vi "GetHandleBySerial.vi"(1 "Serial Number":i16) -> (0 "Handle":i32)   [LabVIEW 2012]
uses:
  Madlib.dll
panel:
  # "Acquires a handle to a specific device. Can be\nused as a subVI."
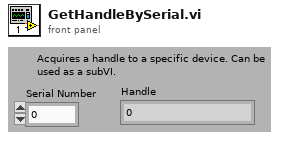
[diagram p1: front panel]
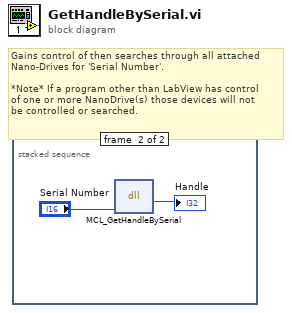
[diagram p0: block diagram]
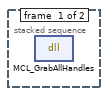
[diagram p2: hidden frame]
diagram:
  # "Gains control of then searches through all attached\nNano-Drives for 'Serial Number'.\n\n*Note* If a program other than LabView has control\nof one or more NanoDrive(s) those devices will not\nbe controlled or searched."
  n1 = stacked-sequence {
    frame #0 {
      n2 = dll-call lib="C:/Users/Labview/Desktop/SRR/Madlib_x64/Labview Examples/MADLib.dll" fn="MCL_GrabAllHandles"() -> ()  [unwired: 4 in, 2 out]
    }
    frame #1 {
      n3 = dll-call lib="C:/Users/Labview/Desktop/SRR/Madlib_x64/Labview Examples/MADLib.dll" fn="MCL_GetHandleBySerial"("serial"="Serial Number") -> (→"Handle":i32)  [unwired: 4 in, 2 out]
    }
  }
